vi "GetCfgMgr.vi"(11 "Attribute.Config in":refnum<class "Attribute.Config.lvclass">) -> (2 "CfgMgr":refnum<class "ConfigManager.lvclass">, 3 "Attribute.Config out":refnum<class "Attribute.Config.lvclass">)   [LabVIEW 2013, in "Attribute.Config.lvclass"]
uses:
  Attribute.Config.lvclass
  <vilib>/LabVIEW Open Source/Configuration Manager/Manager/ConfigManager.lvclass
  Attribute.Config.lvclass/Attribute.Config.ctl
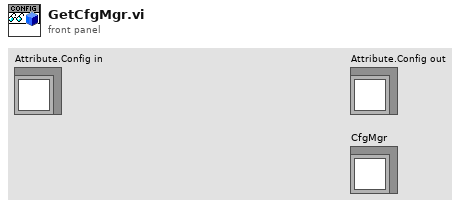
[diagram p1: front panel]
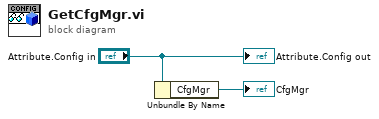
[diagram p0: block diagram]
diagram:
  n1 = Unbundle By Name("Attribute.Config in") -> ("CfgMgr"=→"CfgMgr":refnum<class "ConfigManager.lvclass">)
  "Attribute.Config out" <- "Attribute.Config in"
